vi "Flip and Pad for Picture Control (excel).vi"(3 "bmp to LV? (T)":bool=TRUE, 4 "bitmap info":T1, 5 "BMP bitmap":u8[](array[numeric])) -> (2 "picture bitmap":u8[](array[numeric]))   [LabVIEW 2020, in "NI_ReportGenerationToolkit.lvlib"]
doc: "Transform Windows BMP data to LabVIEW picture bitmap data. Windows gives rows from bottom to top padded out to a 32 bit boundary. LabVIEW expects rows given from top to bottom padded to a 16 bit boundary."
uses:
  <vilib>/addons/_office/NI_ReportGenerationToolkit.lvlib
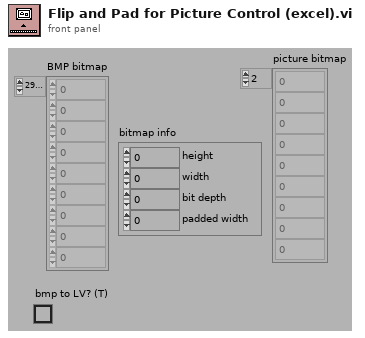
[diagram p1: front panel]
types:
  T1 = cluster{"height":u32, "width":u32, "bit depth":u16, "padded width":u32}
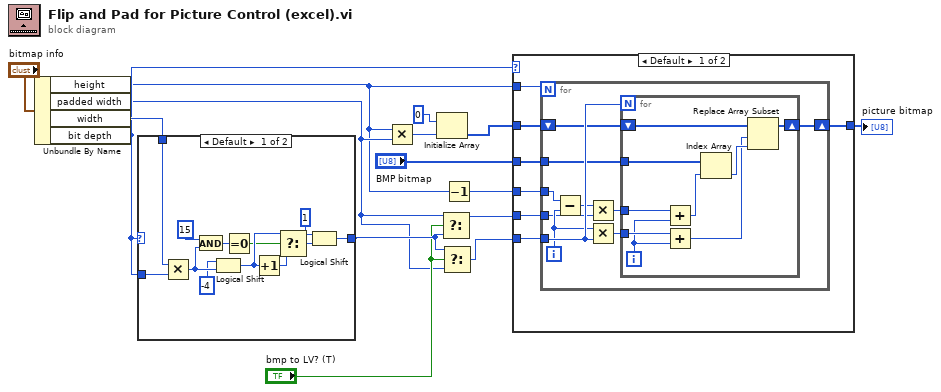
[diagram p0: block diagram]
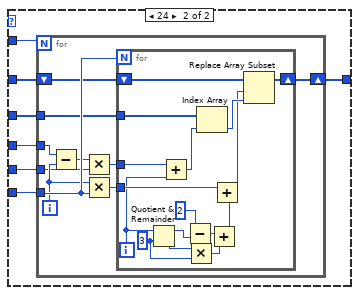
[diagram p2: hidden frame]
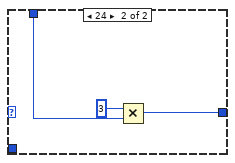
[diagram p3: hidden frame]
diagram:
  n1 = Unbundle By Name("bitmap info") -> ("height"=w2:u32, "padded width"=w3:u32, "width"=w11:u32, "bit depth"=w5:u16)
  n2 = case shown="Default" w5 {
    tunnel: w11 -> [w18 w29]
    tunnel: w5 -> [w17 _]
    tunnel: [w16 w28] -> w9
    frame Default {
      n3 = Multiply(x=w18, y=w17) -> (x*y=w20:u32)
      n4 = And(x=15, y=w20) -> (x .and. y?=w22:u32)
      n5 = Logical Shift(y=-4, x=w20) -> (x << y=w24:u32)
      n6 = Equal To 0?(x=w22) -> (x = 0?=w23:bool)
      n7 = Increment(x=w24) -> (x+1=w25:u32)
      n8 = Select(t=w24, s=w23, f=w25) -> (s? t:f=w27:u32)
      n9 = Logical Shift(y=1, x=w27) -> (x << y=w16:u32)
    }
    frame 24 {
      n10 = Multiply(x=u16 3, y=w29) -> (x*y=w28:u32)
    }
  }
  n11 = Multiply(x=w2, y=w3) -> (x*y=w1:u32)
  n12 = Initialize Array(u8 0, w1) -> (w14:u8[])
  n13 = Select(t=w3, s="bmp to LV? (T)", f=w9) -> (s? t:f=w8:u32)
  n14 = Select(t=w9, s="bmp to LV? (T)", f=w3) -> (s? t:f=w7:u32)
  n15 = Decrement(x=w2) -> (x-1=w15:u32)
  n16 = case shown="Default" w5 {
    tunnel: w15 -> [w37 w63]
    tunnel: w14 -> [w36 w62]
    tunnel: w2 -> [w35 w61]
    tunnel: "BMP bitmap" -> [w34 w60]
    tunnel: w8 -> [w33 w59]
    tunnel: w7 -> [w32 w58]
    tunnel: [w31 w57] -> w4
    frame Default {
      n17 = for {
        N: w35 -> [_]
        shift-right: [w45] -> w31
        shift-left: w36 -> [w46]
        tunnel: w34 -> [w44]
        tunnel: w37 -> [w43]
        tunnel: w33 -> [w38]
        tunnel: w32 -> [w47]
        i -> [w39]
        n18 = Subtract(x=w43, y=w39) -> (x-y=w42:u32)
        n19 = Multiply(x=w42, y=w38) -> (x*y=w41:u32)
        n20 = Multiply(x=w39, y=w47) -> (x*y=w40:u32)
        n21 = for {
          N: w47 -> [_]
          shift-right: [w56] -> w45
          shift-left: w46 -> [w55]
          tunnel: w44 -> [w53]
          tunnel: w41 -> [w52]
          tunnel: w40 -> [w50]
          i -> [w49]
          n22 = Add(x=w52, y=w49) -> (x+y=w51:u32)
          n23 = Add(x=w50, y=w49) -> (x+y=w48:u32)
          n24 = Index Array(array=w53, index=w51) -> (element=w54:u8)
          n25 = Replace Array Subset(array=w55, new element=w54, index=w48) -> (w56:u8[])
        }
      }
    }
    frame 24 {
      n26 = for {
        N: w61 -> [_]
        shift-right: [w71] -> w57
        shift-left: w62 -> [w72]
        tunnel: w60 -> [w70]
        tunnel: w63 -> [w69]
        tunnel: w59 -> [w64]
        tunnel: w58 -> [w73]
        i -> [w65]
        n27 = Subtract(x=w69, y=w65) -> (x-y=w68:u32)
        n28 = Multiply(x=w68, y=w64) -> (x*y=w67:u32)
        n29 = Multiply(x=w65, y=w73) -> (x*y=w66:u32)
        n30 = for {
          N: w73 -> [_]
          shift-right: [w89] -> w71
          shift-left: w72 -> [w88]
          tunnel: w70 -> [w86]
          tunnel: w67 -> [w85]
          tunnel: w66 -> [w83]
          i -> [w81]
          w75 = 3
          n31 = Quotient & Remainder(x=w81, y=w75) -> (x-y*floor(x/y)=w79:i32, floor(x/y)=w76:i32)
          n32 = Add(x=w85, y=w81) -> (x+y=w84:u32)
          n33 = Subtract(x=2, y=w79) -> (x-y=w78:i32)
          n34 = Multiply(x=w76, y=w75) -> (x*y=w74:i32)
          n35 = Index Array(array=w86, index=w84) -> (element=w87:u8)
          n36 = Add(x=w78, y=w74) -> (x+y=w77:i32)
          n37 = Add(x=w83, y=w77) -> (x+y=w82:u32)
          n38 = Replace Array Subset(array=w88, new element=w87, index=w82) -> (w89:u8[])
        }
      }
    }
  }
  "picture bitmap" <- w4
